vi "I2C Write.vi"(5 "EOF":T1, 7 "I2C Channel":u8=1, 8 "Error In":errorcluster, 9 "Data":u8[](array[numeric]), 10 "I2C Slave Address (0)":u8=9, 11 "LINX Resource":T2={"Platform"=enum."LINX", "Interface"=enum."TCP", "LINX Device Config"={"Interface"=enum."TCP", "COM Port"="N/A", "TCP Configuration"={"IP Address"="panicattack", "Port"=6999}, "Device Family"=4, "Device ID"=1, "Device Name"="Raspberry Pi Model B", "TCP Ref"=refnum, "Channels"={"DI Channels"=[2, 3, 4, 7, 8, 9, 10, 11, 14, 15, 17, 18, 22, 23, 24, 25, 27], "DO Channels"=[2, 3, 4, 7, 8, 9, 10, 11, 14, 15, 17, 18, 22, 23, 24, 25, 27], "AI"=[], "AO"=[], "PWM"=[], "QE"=[], "UART"=[0], "I2C 2"=[0, 1], "SPI"=[0], "CAN"=[], "AI Ref (V)"=0.0, "AO Resolution (Bits)"=0, "AO Ref (V)"=0.0}}}) -> (0 "Error Out":errorcluster={"status"=TRUE, "code"=5000, "source"=":\n\nBlinkM.vi >>\nGo To RGB Color Now.vi >>\nI2C Write.vi >>\nI2C Write.vi<ERR>\nAn unknown error occured in LINX I2C Write."}, 3 "LINX Resource":T2={"Platform"=enum."LINX", "Interface"=enum."TCP", "LINX Device Config"={"Interface"=enum."TCP", "COM Port"="N/A", "TCP Configuration"={"IP Address"="panicattack", "Port"=6999}, "Device Family"=4, "Device ID"=1, "Device Name"="Raspberry Pi Model B", "TCP Ref"=refnum, "Channels"={"DI Channels"=[2, 3, 4, 7, 8, 9, 10, 11, 14, 15, 17, 18, 22, 23, 24, 25, 27], "DO Channels"=[2, 3, 4, 7, 8, 9, 10, 11, 14, 15, 17, 18, 22, 23, 24, 25, 27], "AI"=[], "AO"=[], "PWM"=[], "QE"=[], "UART"=[0], "I2C 2"=[0, 1], "SPI"=[0], "CAN"=[], "AI Ref (V)"=0.0, "AO Resolution (Bits)"=0, "AO Ref (V)"=0.0}}})   [LabVIEW 2011, in "LVH-LINX.lvlib"]
doc: "Write data to the specified I2C channel."
uses:
  LVH-LINX.lvlib
  Private/Type Defs/LINX Ref.ctl
  Private/Type Defs/Platform.ctl
  Private/Type Defs/Interface.ctl
  Private/Device/Type Defs/LINX Device Config.ctl
  Private/Device/Type Defs/TCP Config.ctl
  Private/Device/Type Defs/Channels.ctl
  Private/Type Defs/Peripherals/I2C/EOF.ctl
  Private/Type Defs/Peripheral.ctl
  Private/Type Defs/Channel FGV States.ctl
  <vilib>/myRIO/Instrument Drivers/Onboard IO/I2C/typedefs/I2C Transfer Rate.ctl
  <vilib>/myRIO/Instrument Drivers/Onboard IO/I2C/typedefs/I2C Configuration.ctl
  <vilib>/myRIO/Common/Instrument Driver Framework/myRIO v1.0/I2C/typedefs/I2C Channels Enum.ctl
  <vilib>/myRIO/Common/Instrument Driver Framework/Utilities/typedefs/Generic FPGA Reference.ctl
  <vilib>/myRIO/Common/Instrument Driver Framework/Utilities/typedefs/myRIO v1.0 Reference.ctl
  <vilib>/myRIO/Common/Instrument Driver Framework/Utilities/typedefs/Hardware Version Enum.ctl
  <vilib>/myRIO/Common/Instrument Driver Framework/Utilities/typedefs/myRIO Generic Hardware Reference.ctl
  <vilib>/myRIO/Instrument Drivers/Onboard IO/I2C/typedefs/I2C Reference.ctl
  Private/Device/Device.lvlib
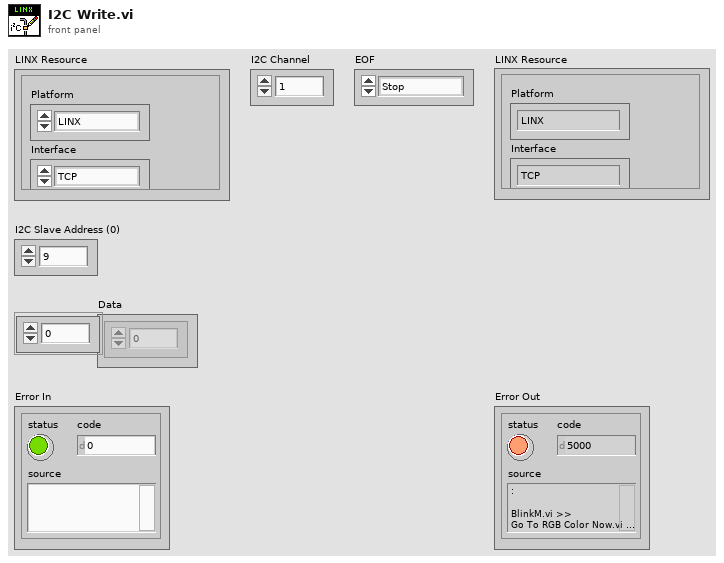
[diagram p1: front panel]
types:
  T1 = typedef "LVH-LINX.lvlib/EOF.ctl" = enum8{"Stop", "Restart", "Restart No Stop", "No Stop"}
  T2 = typedef "LVH-LINX.lvlib/LINX Ref.ctl" = cluster{"Platform":T3, "Interface":T4, "LINX Device Config":T5}
  T3 = typedef "LVH-LINX.lvlib/Platform.ctl" = enum16{"LINX", "myRIO"}
  T4 = typedef "LVH-LINX.lvlib/Interface.ctl" = enum16{"Serial", "TCP"}
  T5 = typedef "LVH-LINX.lvlib/Device.lvlib/LINX Device Config.ctl" = cluster{"Interface":T4, "COM Port":refnum<visa-resource-name>, "TCP Configuration":T6, "Device Family":u8, "Device ID":u8, "Device Name":string, "TCP Ref":refnum<k5>, "Channels":T7}
  T6 = typedef "LVH-LINX.lvlib/Device.lvlib/TCP Config.ctl" = cluster{"IP Address":string, "Port":u16}
  T7 = typedef "LVH-LINX.lvlib/Channels.ctl" = cluster{"DI Channels":u8[], "DO Channels":u8[], "AI":u8[], "AO":u8[], "PWM":u8[], "QE":u8[], "UART":u8[], "I2C 2":u8[], "SPI":u8[], "CAN":u8[], "AI Ref (V)":dbl, "AO Resolution (Bits)":u8, "AO Ref (V)":dbl}
  T8 = typedef "LVH-LINX.lvlib/Peripheral.ctl" = enum8{"DI", "DO", "AI", "AO", "PWM", "QE", "UART", "I2C", "SPI", "CAN"}
  T9 = typedef "LVH-LINX.lvlib/Channel FGV States.ctl" = enum16{"Initialize", "Get", "Set"}
  T10 = typedef "I2C.lvlib/I2C Reference.ctl" = cluster{"myRIO Reference":T11, "I2C Channels Enum":T15, "I2C Configuration":T16}
  T11 = typedef "myRIO Generic Hardware Reference.ctl" = cluster{"myRIO Model":T12, "myRIO Hardware Reference":T13}
  T12 = typedef "Hardware Version Enum.ctl" = enum16{"Unknown", "myRIO-1900", "myRIO-1950"}
  T13 = typedef "myRIO v1.0 Reference.ctl" = cluster{"Generic FPGA Reference":T14, "Allow multiple opens":bool}
  T14 = typedef "Generic FPGA Reference.ctl" = refnum<k20>
  T15 = typedef "I2C Channels Enum.ctl" = enum16{"Not Connected", "A/I2C", "B/I2C"}
  T16 = typedef "I2C.lvlib/I2C Configuration.ctl" = cluster{"I2C Transfer Rate":T17}
  T17 = typedef "I2C.lvlib/I2C Transfer Rate.ctl" = enum16{"Standard Mode (100 kbps)", "Fast Mode (400 kbps)"}
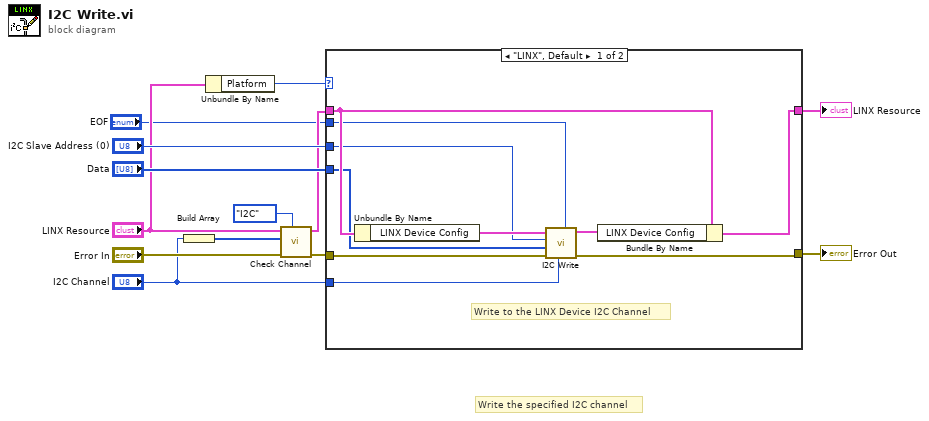
[diagram p0: block diagram]
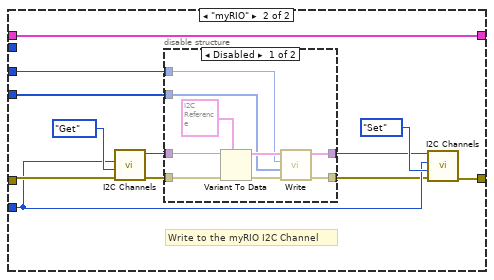
[diagram p2: hidden frame]
diagram:
  # "Write the specified I2C channel"
  n1 = Build Array("I2C Channel") -> (w4:u8[])
  n2 = Unbundle By Name("LINX Resource") -> ("Platform"=w13:T3)
  n3 = call "Check Channel.vi"("Peripheral"=Peripheral."I2C", "Error In"="Error In", "Channels"=w4, "LINX Resource"="LINX Resource") -> ("Error Out"=w6:errorcluster, "LINX Resource"=w2:T2)  [unwired: 5 in, 1 out]
  n4 = case shown="\"LINX\", Default" w13 {
    tunnel: w6 -> [w20 w31]
    tunnel: w2 -> [w23 w35]
    tunnel: [w21 w34] -> w12
    tunnel: [w22 w35] -> w11
    tunnel: "I2C Channel" -> [w17 w30]
    tunnel: "Data" -> [w15 w26]
    tunnel: "I2C Slave Address (0)" -> [w16 w25]
    tunnel: "EOF" -> [w14 _]
    frame "LINX", Default {
      # "Write to the LINX Device I2C Channel"
      n5 = Unbundle By Name(w23) -> ("LINX Device Config"=w18:T5)
      n6 = call "I2C Write.vi"("EOF"=w14, "I2C Channel (0)"=w17, "Error In"=w20, "Data"=w15, "I2C Slave Address"=w16, "LINX Device Config"=w18) -> ("Error Out"=w21:errorcluster, "LINX Device Config"=w19:T5)  [unwired: 4 in]
      n7 = Bundle By Name(cluster=w23, "LINX Device Config"=w19) -> (w22:T2)
    }
    frame "myRIO" {
      # "Write to the myRIO I2C Channel"
      n8 = call "I2C Channels.vi"("Error In"=w31, "Channel State"=Channel_FGV_States."Get", "Channel Number"=w30) -> ("Error Out"=w29:errorcluster, "I2C Channel"=w27:variant)  [unwired: 7 in]
      n9 = disable-structure shown="Disabled" {
        disable-tunnel: w29 -> [w41 _]
        disable-tunnel: [w40 _] -> w28
        disable-tunnel: w27 -> [w39 _]
        disable-tunnel: w26 -> [w38 _]
        disable-tunnel: w25 -> [w37 _]
        disable-tunnel: [w36 _] -> w24
        frame Disabled {
          n10 = Variant To Data(error in=w41, type=T10 {"myRIO Reference"={"myRIO Model"=enum."Unknown", "myRIO Hardware Reference"={"Generic FPGA Reference"=refnum, "Allow multiple opens"=FALSE}}, "I2C Channels Enum"=enum."Not Connected", "I2C Configuration"={"I2C Transfer Rate"=enum."Standard Mode (100 kbps)"}}, Variant=w39) -> (data=w44:T10, error out=w42:errorcluster)
          n11 = call <vilib>:"Write.vi"("error in (no error)"=w42, "Bytes to Write"=w38, "Slave Address (7-bit)"=w37, "I2C Ref In"=w44) -> ("error out"=w40:errorcluster, "I2C Ref Out"=w36:T10)  [unwired: 6 in]
        }
        frame Enabled {
        }
      }
      n12 = call "I2C Channels.vi"("Error In"=w28, "Channel State"=Channel_FGV_States."Set", "Channel Number"=w30, "I2C Channel"=w24) -> ("Error Out"=w34:errorcluster)  [unwired: 6 in, 1 out]
    }
  }
  "Error Out" <- w12
  "LINX Resource" <- w11
